vi "Add VI to Owner Library or Class.vi"(8 "error in":errorcluster, 10 "Reference of newly created VI":refnum<vi>, 11 "Owner Reference (Library or Class)":refnum<vi>) -> (0 "error out":errorcluster)   [LabVIEW 2020]
doc: "<add doc>"
panel:
  # "Development\ncontrols/indicators useful for development and testing, but which are not outputs of the VI"
  # "Input\nInputs to the VI"
  # "Output\nOutputs of the VI"
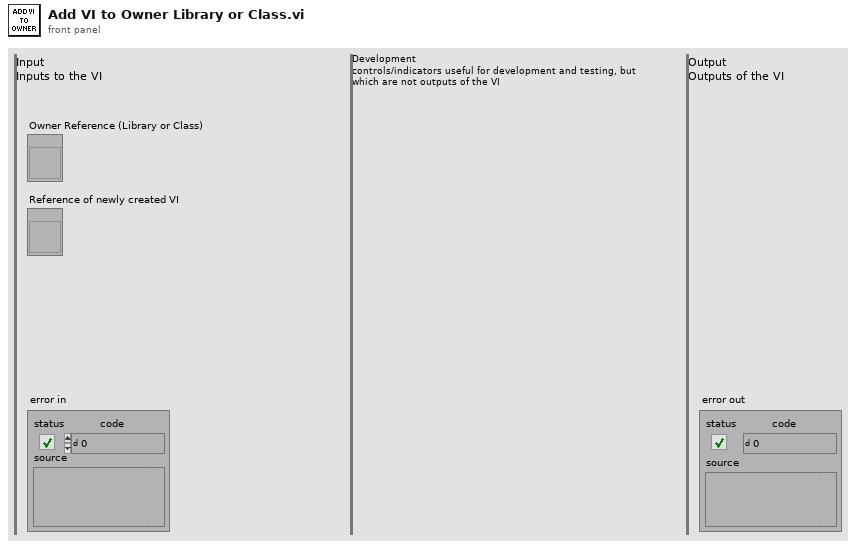
[diagram p1: front panel]
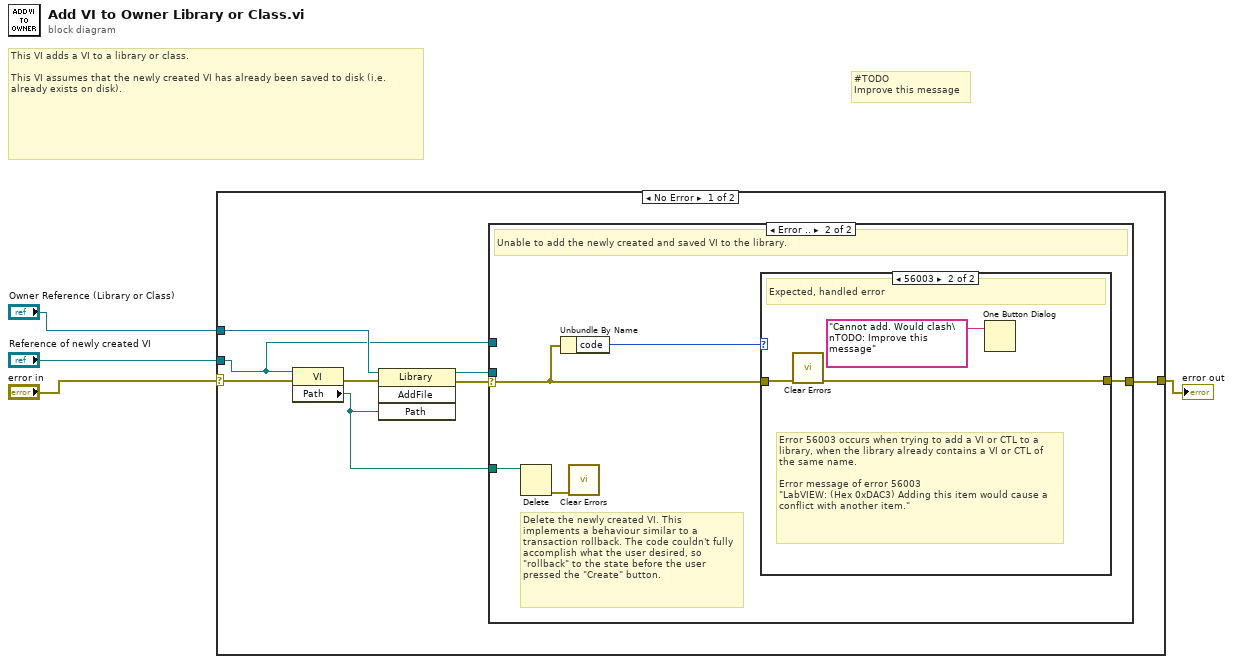
[diagram p0: block diagram]
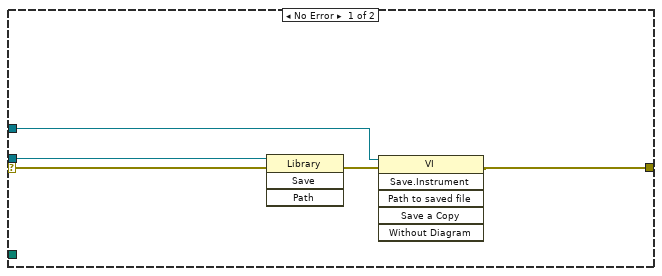
[diagram p2: hidden frame]
diagram:
  # "#TODO\nImprove this message"
  # "This VI adds a VI to a library or class.\n\nThis VI assumes that the newly created VI has already been saved to disk (i.e. already exists on disk)."
  n1 = case shown="No Error" "error in" {
    selector: "error in" -> [w10 w27]
    tunnel: [w9 w27] -> w3
    tunnel: "Owner Reference (Library or Class)" -> [w8 _]
    tunnel: "Reference of newly created VI" -> [w6 _]
    frame No Error {
      n2 = property class="VI"(reference=w6, error in=w10) -> (error out=w7:errorcluster, "Path"=w5:path)  [unwired: 1 out]
      n3 = invoke class="Library" method="AddFile"(reference=w8, error in=w7, "Path"=w5) -> (reference out=w11:refnum<vi>, error out=w12:errorcluster)  [unwired: 1 in, 2 out]
      n4 = case shown="Error .." w12 {
        selector: w12 -> [w17 w20]
        tunnel: w11 -> [w15 _]
        tunnel: [w14 w21] -> w9
        tunnel: w6 -> [w13 _]
        tunnel: w5 -> [_ w19]
        frame No Error {
          n5 = invoke class="Library" method="Save"(reference=w15, error in=w17) -> (error out=w16:errorcluster)  [unwired: 2 in, 3 out]
          n6 = invoke class="VI" method="Save.Instrument"(reference=w13, error in=w16) -> (error out=w14:errorcluster)  [unwired: 4 in, 5 out]
        }
        frame Error {
          # "Delete the newly created VI. This implements a behaviour similar to a transaction rollback. The code couldn't fully accomplish what the user desired, so \"rollback\" to the state before the user pressed the \"Create\" button."
          # "Unable to add the newly created and saved VI to the library."
          n7 = Delete(path (use dialog)=w19) -> (error out=w18:errorcluster)  [unwired: 4 in, 2 out]
          n8 = Unbundle By Name(w20) -> ("code"=w22:i32)
          n9 = call <vilib>:"Clear Errors.vi"("error in (no error)"=w18) -> ()  [unwired: 5 in, 2 out]
          n10 = case shown="56003" w22 {
            tunnel: w20 -> [w23 w26]
            tunnel: [w23 w24] -> w21
            frame Default {
              # "Do nothing. The error will be handled downstream."
              # "Unexpected error"
            }
            frame 56003 {
              # "Error 56003 occurs when trying to add a VI or CTL to a library, when the library already contains a VI or CTL of the same name.\n\nError message of error 56003\n\"LabVIEW: (Hex 0xDAC3) Adding this item would cause a conflict with another item.\""
              # "Expected, handled error"
              n11 = call <vilib>:"Clear Errors.vi"("error in (no error)"=w26) -> ("error out"=w24:errorcluster)  [unwired: 5 in, 1 out]
              n12 = One Button Dialog(message="Cannot add. Would clash\nTODO: Improve this message") -> ()  [unwired: 1 in, 1 out]
            }
          }
        }
      }
    }
    frame Error {
    }
  }
  "error out" <- w3
